vi "Backlash correction.vi"(0 "Lifter_motor in":refnum<class "Lifter_motor.lvclass">, 5 "Direction is chaged":bool, 11 "error in (no error)":errorcluster) -> (4 "Lifter_motor out":refnum<class "Lifter_motor.lvclass">, 15 "error out":errorcluster)   [LabVIEW 2019, in "Lifter_motor.lvclass"]
uses:
  Lifter_motor.lvclass
  Lifter_motor.lvclass/Lifter_motor.ctl
panel:
  out "Backlash correction (on/off)":bool
  out "New direction":bool
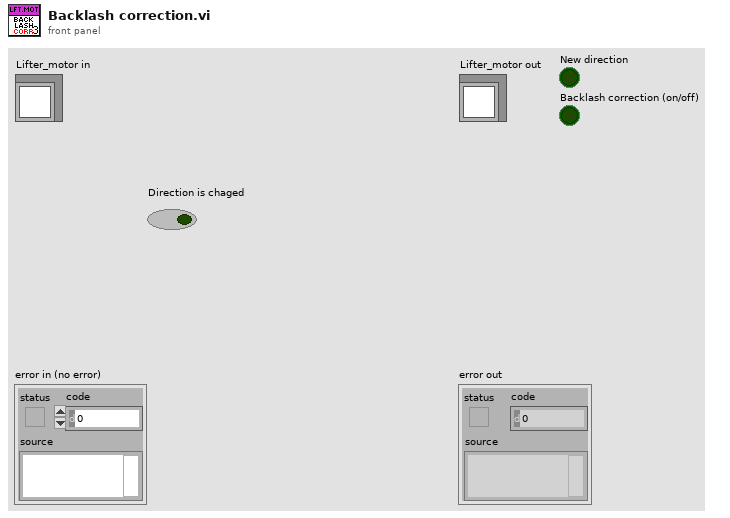
[diagram p1: front panel]
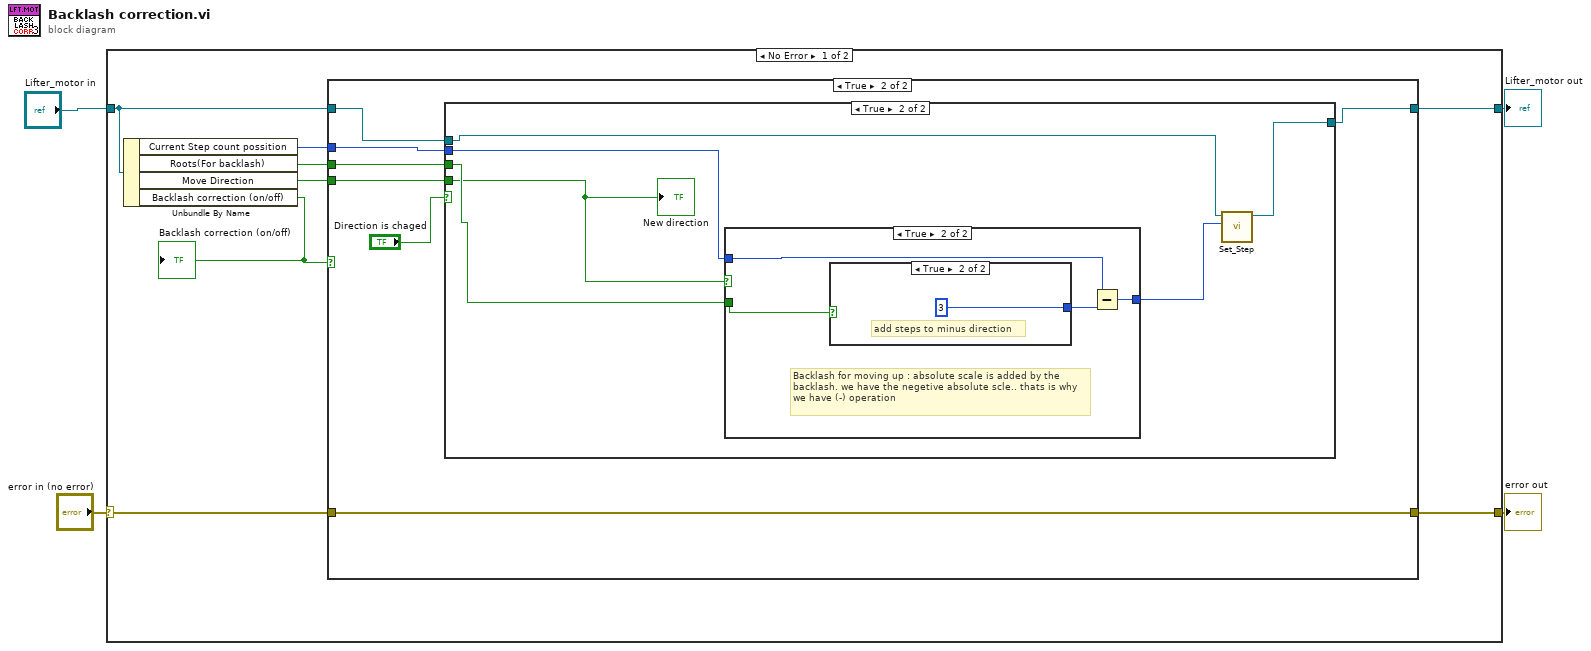
[diagram p0: block diagram]
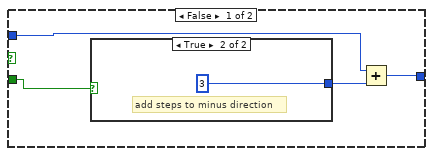
[diagram p4: hidden frame]
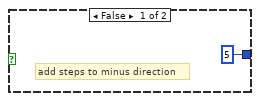
[diagram p5: hidden frame]
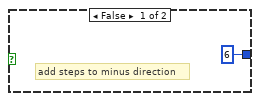
[diagram p6: hidden frame]
diagram:
  n1 = case shown="No Error" "error in (no error)" {
    selector: "error in (no error)" -> [w11 w42]
    tunnel: [w10 w42] -> w3
    tunnel: [w12 w41] -> w1
    tunnel: "Lifter_motor in" -> [w7 w41]
    frame No Error {
      n2 = Unbundle By Name(w7) -> ("Current Step count possition"=w9:i32, "Roots(For backlash)"=w8:bool, "Move Direction"=w6:bool, "Backlash correction (on/off)"=w5:bool)
      "Backlash correction (on/off)" <- w5
      n3 = case shown="True" w5 {
        tunnel: w7 -> [w14 w20]
        tunnel: [w14 w19] -> w12
        tunnel: w11 -> [w13 w18]
        tunnel: [w13 w18] -> w10
        tunnel: w9 -> [_ w17]
        tunnel: w8 -> [_ w16]
        tunnel: w6 -> [_ w15]
        frame False {
        }
        frame True {
          n4 = case shown="True" "Direction is chaged" {
            tunnel: w20 -> [w22 w24]
            tunnel: [w22 w28] -> w19
            tunnel: w17 -> [_ w26]
            tunnel: w16 -> [_ w25]
            tunnel: w15 -> [_ w23]
            frame False {
            }
            frame True {
              n5 = case shown="True" w23 {
                tunnel: w25 -> [w32 w38]
                tunnel: w26 -> [w30 w37]
                tunnel: [w29 w35] -> w27
                frame False {
                  n6 = case shown="True" w32 {
                    tunnel: [5 ("y") 3 ("y")] -> w31
                    frame False {
                      # "add steps to minus direction"
                    }
                    frame True {
                      # "add steps to minus direction"
                    }
                  }
                  n7 = Add(x=w30, y=w31) -> (x+y=w29:i32)
                }
                frame True {
                  # "Backlash for moving up : absolute scale is added by the backlash. we have the negetive absolute scle.. thats is why we have (-) operation"
                  n8 = case shown="True" w38 {
                    tunnel: [6 ("y") 3 ("y")] -> w36
                    frame False {
                      # "add steps to minus direction"
                    }
                    frame True {
                      # "add steps to minus direction"
                    }
                  }
                  n9 = Subtract(x=w37, y=w36) -> (x-y=w35:i32)
                }
              }
              n10 = call "Set_Step.vi"("Set_stepcount"=w27, "Lifter_motor in"=w24) -> ("Lifter_motor out"=w28:refnum<class "Lifter_motor.lvclass">)  [unwired: 8 in, 1 out]
              "New direction" <- w23
            }
          }
        }
      }
    }
    frame Error {
    }
  }
  "error out" <- w3
  "Lifter_motor out" <- w1
